vi "testCameraFloor.vi"() -> ()   [LabVIEW 2018]
uses:
  <vilib>/userdefined/High Color/IMAQdx.ctl
  vision/Vision info.vi
  <vilib>/vision/driver/NI_Vision_Acquisition_Software.lvlib
  <resource>/objmgr/imaqdx.rc
panel:
  in  "no":i32
  in  "yes":i32
  out "Image":T1(plugin-control)
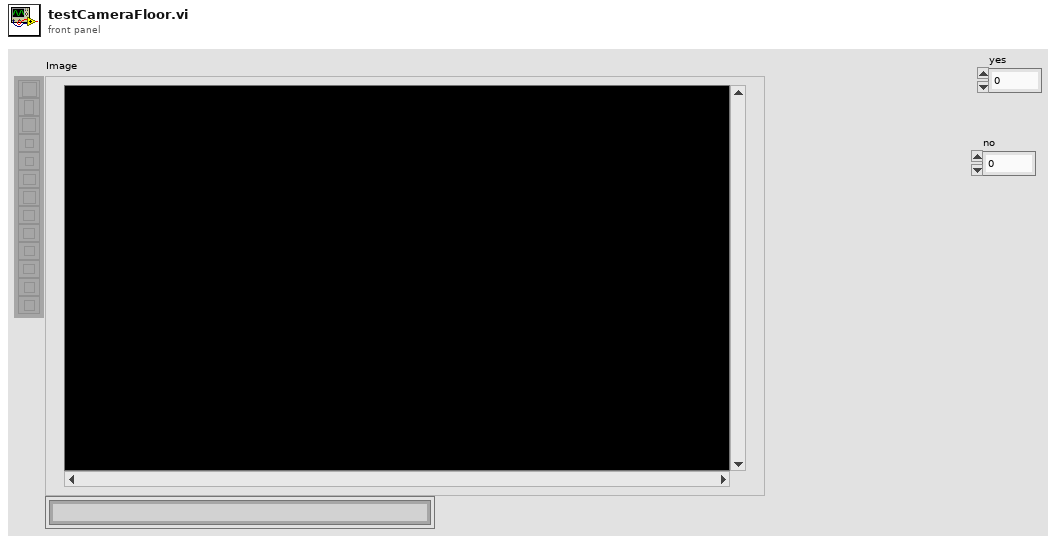
[diagram p1: front panel]
types:
  T1 = typedef "IMAQ Image.ctl" = refnum<image>
  T2 = typedef "IMAQdx.ctl" = refnum<k21>
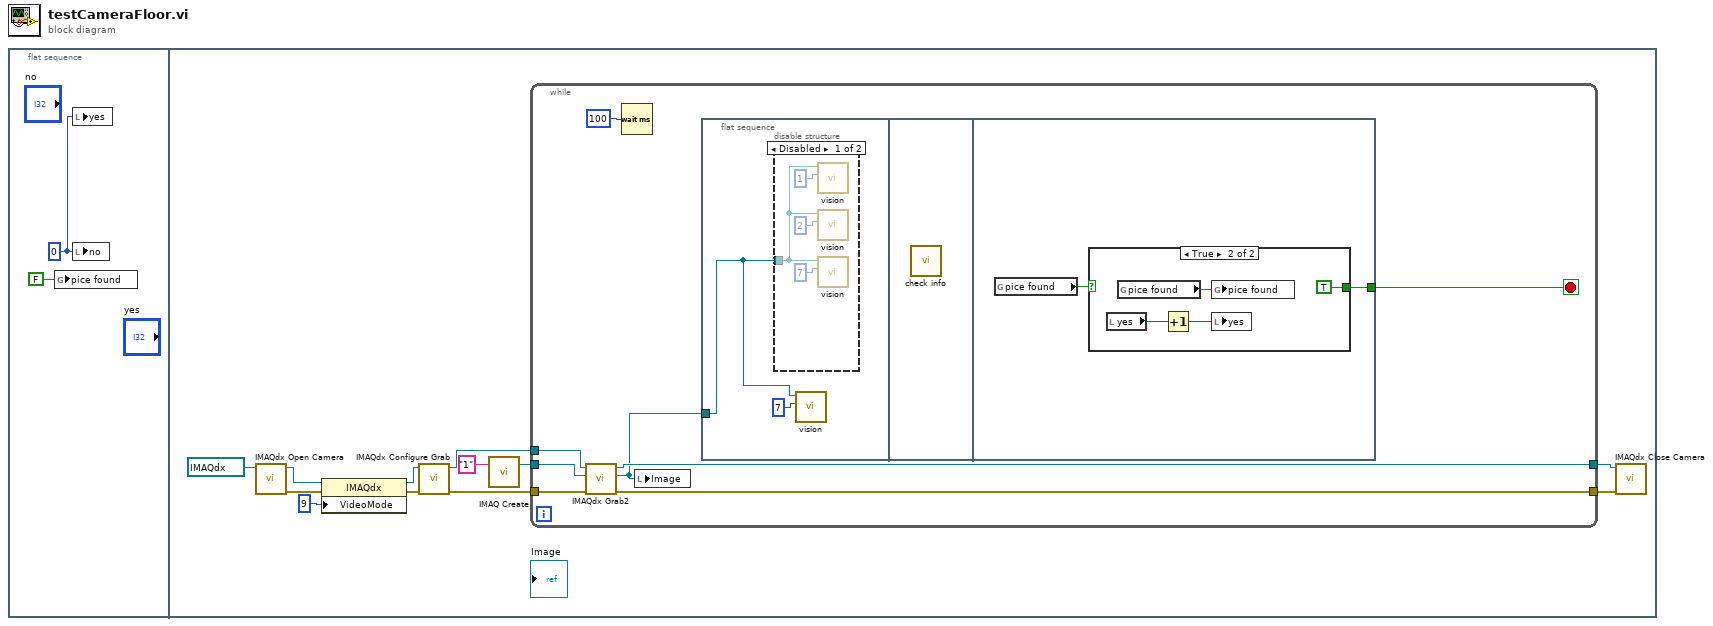
[diagram p0: block diagram]
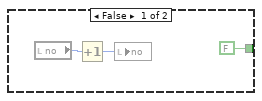
[diagram p3: hidden frame]
diagram:
  n1 = flat-sequence {
    frame #0 {
      w2 = 0 ("yes")
      n2 = global write "Vision info.vi" "pice found"(FALSE ("pice found")) -> ()
      n3 = local write "yes"(w2) -> ()
      n4 = local write "no"(w2) -> ()
    }
    frame #1 {
      n5 = call <vilib>:"IMAQdx Open Camera.vi"("Session In"=T2 "cam0") -> ("error out"=w6:errorcluster, "Session Out"=w7:T2)  [unwired: 9 in]
      n6 = property class="IMAQdx"(reference=w7, error in=w6, "VideoMode"=u32 9) -> (reference out=w4:T2, error out=w5:errorcluster)
      n7 = call <vilib>:"IMAQdx Configure Grab.vi"("error in"=w5, "Session In"=w4) -> ("error out"=w13:errorcluster, "Session Out"=w12:T2)  [unwired: 8 in]
      n8 = call "IMAQ Create"("Image Name"="1") -> ("New Image"=w10:T1)  [unwired: 4 in, 1 out]
      n9 = while {
        tunnel: w13 -> [w22]
        tunnel: w12 -> [w21]
        tunnel: [w20] -> w11
        tunnel: w10 -> [w19]
        tunnel: [w18] -> w8
        stop <- w15 stop-if-true
        n10 = call <vilib>:"IMAQdx Grab2.vi"("error in"=w22, "Image In"=w19, "Session In"=w21) -> ("error out"=w18:errorcluster, "Image Out"=w16:T1, "Session Out"=w20:T2)  [unwired: 5 in, 1 out]
        n11 = Wait (ms)(milliseconds to wait=u32 100) -> ()  [unwired: 1 out]
        n12 = local write "Image"(w16) -> ()
        n13 = flat-sequence {
          tunnel: w16 -> [w23]
          tunnel: [w29] -> w15
          frame #0 {
            n14 = disable-structure shown="Disabled" {
              disable-tunnel: w23 -> [w25 _]
              frame Disabled {
                n15 = call "vision.vi"("Color Plane"=1, "Refnum in"=w25) -> ()  [unwired: 10 in]
                n16 = call "vision.vi"("Color Plane"=2, "Refnum in"=w25) -> ()  [unwired: 10 in]
                n17 = call "vision.vi"("Color Plane"=7, "Refnum in"=w25) -> ()  [unwired: 10 in]
              }
              frame Enabled {
              }
            }
            n18 = call "vision.vi"("Image 3"=w23, "Color Plane"=7) -> ()  [unwired: 9 in]
          }
          frame #1 {
            n19 = call "check info.vi"() -> ()  [unwired: 12 in]
          }
          frame #2 {
            n20 = global read "Vision info.vi" "pice found"() -> (w30:bool)
            n21 = case shown="True" w30 {
              tunnel: [FALSE TRUE] -> w29
              frame False {
                n22 = local read "no"() -> (w32:i32)
                n23 = Increment(x=w32) -> (x+1=w33:i32)
                n24 = local write "no"(w33) -> ()
              }
              frame True {
                n25 = local read "yes"() -> (w36:i32)
                n26 = global read "Vision info.vi" "pice found"() -> (w34:bool)
                n27 = Increment(x=w36) -> (x+1=w37:i32)
                n28 = global write "Vision info.vi" "pice found"(w34) -> ()
                n29 = local write "yes"(w37) -> ()
              }
            }
          }
        }
      }
      n30 = call <vilib>:"IMAQdx Close Camera.vi"("error in"=w8, "Session In"=w11) -> ()  [unwired: 9 in, 1 out]
    }
  }
